vi "Desktop Main.vi"() -> ()   [LabVIEW 2021]
doc: "Demonstrates the use of Transmission Control Protocol (TCP) and meta data to transimit messages from the host computer to the myRIO."
panel:
  in  "LED":bool[](array[boolean])=[FALSE, FALSE, FALSE, FALSE]
  out "error out":errorcluster
  in  "Meta Data":string[](array[string])=["LED Status"]
  in  "Stop":bool
  # "Overview: Demonstrates the use of Transmission Control Protocol (TCP) and meta data to transimit  messages from the host computer to the myRIO.\nInstructions:\n1. Run this VI.\n2. Open RT Main.vi and follow its front panel instructions.\n3. Change the value of LED on this VI and observe the LEDs on the myRIO device and the value of LED Status on the RT Main.vi.\n4. Click Stop to stop this VI. Stopping this VI also terminates the running of RT Main.vi."
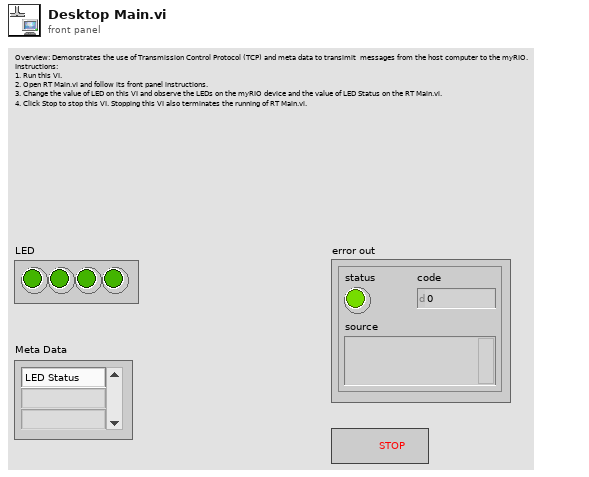
[diagram p1: front panel]
types:
  T1 = typedef "Connection Info.ctl" = cluster{"connection ID":refnum<k5>, "Meta data":string[]}
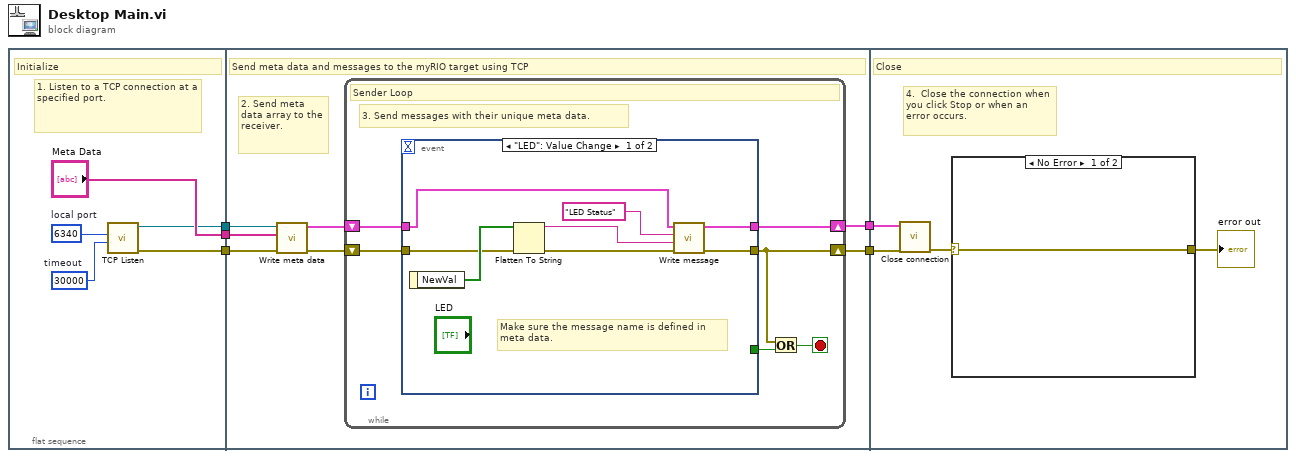
[diagram p0: block diagram]
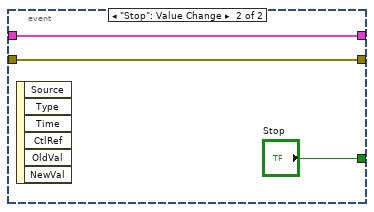
[diagram p2: hidden frame]
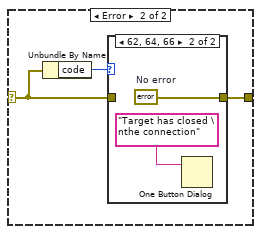
[diagram p3: hidden frame]
diagram:
  n1 = flat-sequence {
    tunnel: ["Meta Data"] -> w3
    tunnel: [w9] -> w2
    tunnel: [w8] -> w1
    tunnel: [w17] -> w5
    tunnel: [w16] -> w4
    tunnel: w3 -> [w13]
    tunnel: w2 -> [w12]
    tunnel: w1 -> [w11]
    tunnel: w5 -> [w38]
    tunnel: w4 -> [w37]
    frame #0 {
      w6 = u16 6340  # local port
      w7 = 30000  # timeout
      # "1. Listen to a TCP connection at a specified port."
      # "Initialize"
      n2 = call <vilib>:"TCP Listen.vi"("timeout ms (wait forever: -1)"=w7, "port"=w6) -> ("error out"=w8:errorcluster, "connection ID"=w9:refnum<k5>)  [unwired: 2 in, 6 out]
    }
    frame #1 {
      # "2. Send meta data array to the receiver."
      # "Send meta data and messages to the myRIO target using TCP"
      n3 = call "Write meta data.vi"("error in"=w11, "Meta data"=w13, "connection ID"=w12) -> ("error out"=w14:errorcluster, "Connection Info"=w15:T1)  [unwired: 7 in]
      n4 = while {
        shift-right: [w21] -> w16
        shift-left: w14 -> [w19]
        shift-right: [w23] -> w17
        shift-left: w15 -> [w20]
        stop <- w22 stop-if-true
        # "3. Send messages with their unique meta data."
        # "Sender Loop"
        n5 = event shown="[0] \"LED\": Value Change" {
          selector: _ -> [_ _]
          dyn-events: _ -> [_ _]
          timeout: _ -> [_ _]
          tunnel: [w31 w33] -> w23
          tunnel: [w28 w32] -> w21
          tunnel: w20 -> [w27 w33]
          tunnel: w19 -> [w25 w32]
          tunnel: [_ "Stop"] -> w18
          event "LED": Value Change {
            # "Make sure the message name is defined in \nmeta data."
            n6 = event-data() -> ("NewVal"=w26:bool[])  [unwired: 1 in]
            n7 = Flatten To String(anything=w26, error in (no error)=w25) -> (data string=w30:string, error out=w24:errorcluster)  [unwired: 3 out]
            n8 = call "Write message.vi"("error in"=w24, "Value"=w30, "Message Name"="LED Status" ("Name"), "Connection Info"=w27) -> ("error out"=w28:errorcluster, "Connection Info out"=w31:T1)  [unwired: 6 in]
          }
          event "Stop": Value Change {
            n9 = event-data() -> ()  [unwired: 1 in, 6 out]
          }
        }
        n10 = Or(x=w21, y=w18) -> (x .or. y?=w22:bool)
      }
    }
    frame #2 {
      # "4.  Close the connection when you click Stop or when an error occurs."
      # "Close"
      n11 = call "Close connection.vi"("error in"=w37, "Connection Info"=w38) -> ("error out"=w36:errorcluster)  [unwired: 8 in, 1 out]
      n12 = case shown="No Error" w36 {
        selector: w36 -> [w39 w40]
        tunnel: [w39 w41] -> w35
        frame No Error {
        }
        frame Error {
          n13 = Unbundle By Name(w40) -> ("code"=w42:i32)
          n14 = case shown="62, 64, 66" w42 {
            tunnel: w40 -> [w43 _]
            tunnel: [w43 w44] -> w41
            frame Default {
            }
            frame 62, 64, 66 {
              w44 = errorcluster {"status"=FALSE, "code"=0, "source"=""}  # No error
              n15 = One Button Dialog(message="Target has closed \nthe connection") -> ()  [unwired: 1 in, 1 out]
            }
          }
        }
      }
      "error out" <- w35
    }
  }
